vi "EnterDUTInfo.vi"(0 "Enable":bool=TRUE, 5 "error in (no error)":errorcluster, 6 "InputData":string="Enter DUT INFO", 7 "Leidos_sn(t)":bool) -> (10 "DUT INFO":string, 12 "MFR":string, 13 "Desc":string, 14 "SN":string, 15 "LotID":string, 16 "Revision":string, 17 "RaGE PN":string, 18 "OK":bool, 19 "error out":errorcluster)   [LabVIEW 2018]
doc: "Displays a standard dialog box that prompts users to enter information, such as a user name and password.\n--------------------\n\nThis Express VI is configured as follows:\n\nMessage to Display to the User:Enter DUT INFO\nThe inputs are: \nText Entry Box: RaGE PN\nText Entry Box: Revision\nText Entry Box: LotID\nText Entry Box: SN\nText Entry Box: Desc\nText Entry Box: MFR"
panel:
  in  "ESN":string caption="SN"
  out "ESN":string caption="SN"
  in  "MFR":string
  in  "Desc":string
  in  "SN":string
  in  "LotID":string
  in  "Revision":string
  in  "RaGE PN":string
  out "String":string="Enter DUT INFO"
  in  "Cancel":bool
  in  "OK2":bool
  in  "OK1":bool
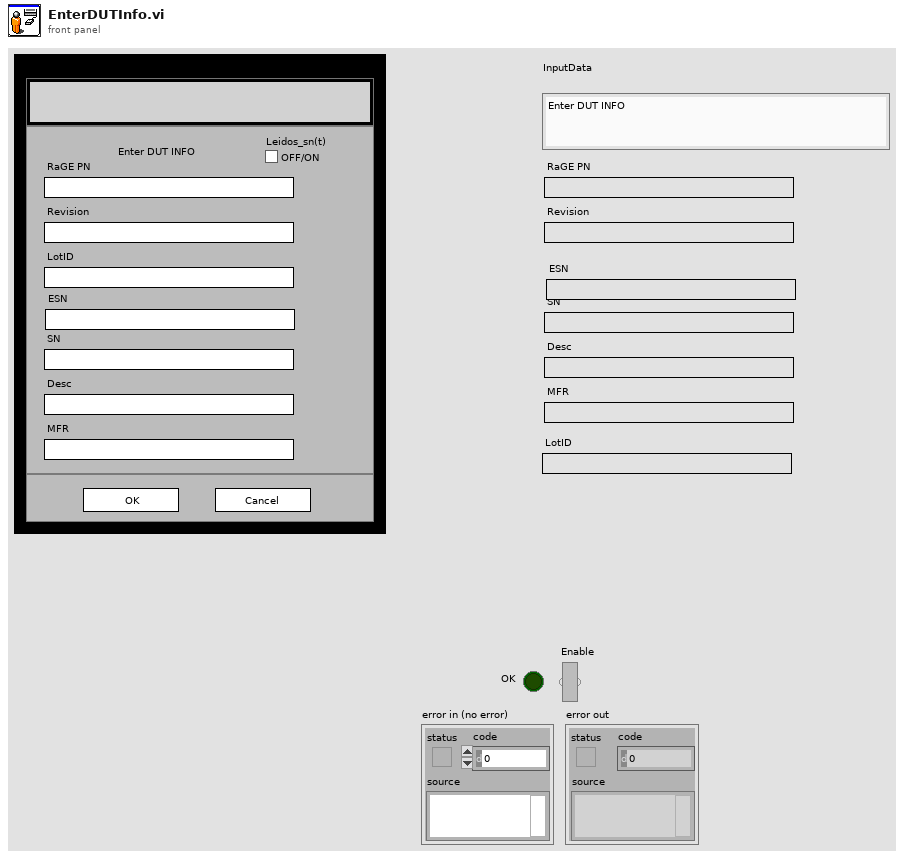
[diagram p1: front panel]
types:
  T1 = enum8{"Enabled", "Disabled", "Disabled and Grayed Out"}
  T2 = cluster{"Input Name":string, "Input Data Type":i32}[]
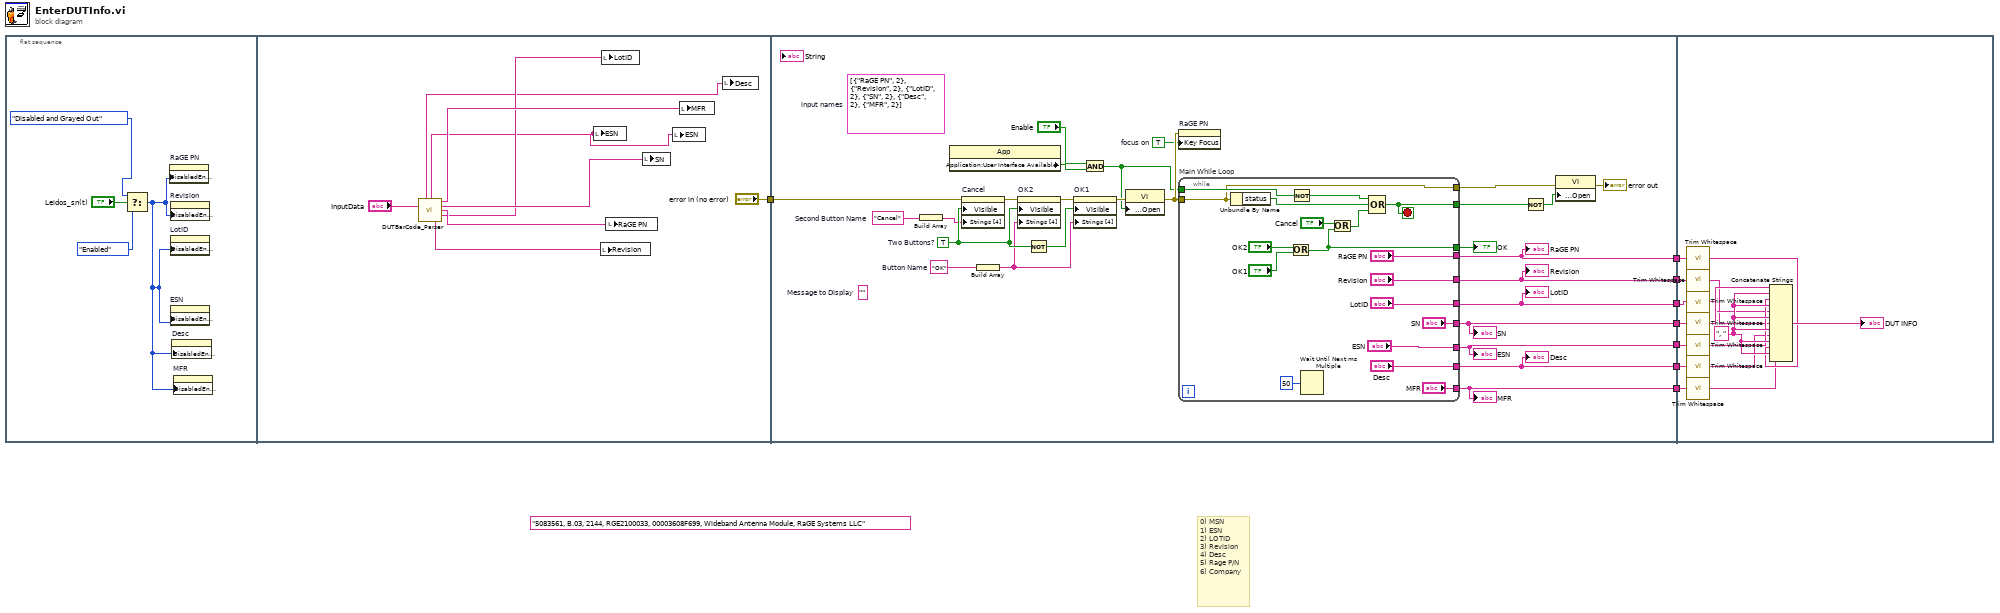
[diagram p0: block diagram]
diagram:
  (unwired) "5083561, B.03, 2144, RGE2100033, 00003608F699, Wideband Antenna Module, RaGE Systems LLC" ("Bar Code")
  # "0) MSN\n1) ESN\n2) LOTID\n3) Revision \n4) Desc\n5) Rage P/N\n6) Company"
  n1 = flat-sequence {
    tunnel: ["error in (no error)"] -> w8
    tunnel: w8 -> [w29]
    tunnel: [w28] -> w7
    tunnel: [w27] -> w6
    tunnel: [w23] -> w5
    tunnel: [w26] -> w4
    tunnel: [w25] -> w3
    tunnel: [w24] -> w2
    tunnel: [w22] -> w1
    tunnel: w7 -> [w82]
    tunnel: w6 -> [w81]
    tunnel: w5 -> [w80]
    tunnel: w4 -> [w79]
    tunnel: w3 -> [w77]
    tunnel: w2 -> [w75]
    tunnel: w1 -> [w74]
    frame #0 {
      n2 = Select(t=T1."Disabled and Grayed Out" ("Disabled"), s="Leidos_sn(t)", f=T1."Enabled" ("Disabled")) -> (s? t:f=w11:T1)
      n3 = property on="RaGE PN" class="Str"("DisabledEnum"=w11) -> ()  [unwired: 2 in, 2 out]
      n4 = property on="Revision" class="Str"("DisabledEnum"=w11) -> ()  [unwired: 2 in, 2 out]
      n5 = property on="LotID" class="Str"("DisabledEnum"=w11) -> ()  [unwired: 2 in, 2 out]
      n6 = property on="ESN" class="Str"("DisabledEnum"=w11) -> ()  [unwired: 2 in, 2 out]
      n7 = property on="Desc" class="Str"("DisabledEnum"=w11) -> ()  [unwired: 2 in, 2 out]
      n8 = property on="MFR" class="Str"("DisabledEnum"=w11) -> ()  [unwired: 2 in, 2 out]
    }
    frame #1 {
      n9 = call "DUTBarCode_Parser.vi"("DUT INFO"="InputData") -> ("Desc"=w14:string, "BC_ESN"=w13:string, "Company"=w19:string, "BC_MSN"=w18:string, "Rage PN"=w17:string, "LotID"=w15:string, "Revision"=w16:string)  [unwired: 5 in, 3 out]
      n10 = local write "ESN"(w13) -> ()
      n11 = local write "Revision"(w16) -> ()
      n12 = local write "LotID"(w15) -> ()
      n13 = local write "RaGE PN"(w17) -> ()
      n14 = local write "SN"(w18) -> ()
      n15 = local write "ESN"(w13) -> ()
      n16 = local write "MFR"(w19) -> ()
      n17 = local write "Desc"(w14) -> ()
    }
    frame #2 {
      w30 = TRUE  # focus on
      (unwired) T2 [{"Input Name"="RaGE PN", "Input Data Type"=2}, {"Input Name"="Revision", "Input Data Type"=2}, {"Input Name"="LotID", "Input Data Type"=2}, {"Input Name"="SN", "Input Data Type"=2}, {"Input Name"="Desc", "Input Data Type"=2}, {"Input Name"="MFR", "Input Data Type"=2}]  # input names
      w40 = "Cancel"  # Second Button Name
      w38 = "OK"  # Button Name
      (unwired) ""  # Message to Display
      w48 = TRUE  # Two Buttons?
      n18 = Build Array(w40) -> (w41:string[])
      n19 = property class="App"() -> ("Application:User Interface Available"=w31:bool)  [unwired: 2 in, 2 out]
      n20 = property on="Cancel" class="Bool"(error in=w29, "Visible"=w48, "Strings [4]"=w41) -> (error out=w45:errorcluster)  [unwired: 1 in, 1 out]
      n21 = Build Array(w38) -> (w39:string[])
      n22 = property on="OK2" class="Bool"(error in=w45, "Visible"=w48, "Strings [4]"=w39) -> (error out=w44:errorcluster)  [unwired: 1 in, 1 out]
      n23 = Not(x=w48) -> (.not. x?=w46:bool)
      n24 = property on="OK1" class="Bool"(error in=w44, "Visible"=w46, "Strings [4]"=w39) -> (error out=w37:errorcluster)  [unwired: 1 in, 1 out]
      n25 = And(x="Enable", y=w31) -> (x .and. y?=w32:bool)
      n26 = property class="VI"(error in=w37, "Front Panel Window:Open"=w32) -> (error out=w36:errorcluster)  [unwired: 1 in, 1 out]
      n27 = property on="RaGE PN" class="Str"(error in=w36, "Key Focus"=w30) -> ()  [unwired: 1 in, 2 out]
      n28 = while "Main While Loop" {
        tunnel: [w63] -> w47
        tunnel: w32 -> [w61]
        tunnel: [w59] -> w42
        tunnel: w36 -> [w58]
        tunnel: [w58] -> w35
        tunnel: ["RaGE PN"] -> w28
        tunnel: ["Revision"] -> w27
        tunnel: ["LotID"] -> w24
        tunnel: ["SN"] -> w22
        tunnel: ["Desc"] -> w26
        tunnel: ["MFR"] -> w25
        tunnel: ["ESN"] -> w23
        stop <- w59 stop-if-true
        n29 = Unbundle By Name(w58) -> ("status"=w56:bool)
        n30 = Or(x="OK2", y="OK1") -> (x .or. y?=w63:bool)
        n31 = Not(x=w61) -> (.not. x?=w60:bool)
        n32 = Wait Until Next ms Multiple(millisecond multiple=u32 50) -> ()  [unwired: 1 out]
        n33 = Or(x="Cancel", y=w63) -> (x .or. y?=w57:bool)
        n34 = Compound Arithmetic op=OR(w60, w56, w57) -> (w59:bool)
      }
      "OK" <- w47
      "RaGE PN" <- w28
      "Revision" <- w27
      "LotID" <- w24
      "SN" <- w22
      "Desc" <- w26
      "MFR" <- w25
      "ESN" <- w23
      n35 = Not(x=w42) -> (.not. x?=w43:bool)
      n36 = property class="VI"(error in=w35, "Front Panel Window:Open"=w43) -> (error out=→"error out":errorcluster)  [unwired: 1 in, 1 out]
    }
    frame #3 {
      w78 = ", " ("string")
      n37 = call <vilib>:"Trim Whitespace.vi"("string"=w82) -> ("trimmed string"=w68:string)  [unwired: 1 in]
      n38 = call <vilib>:"Trim Whitespace.vi"("string"=w81) -> ("trimmed string"=w70:string)  [unwired: 1 in]
      n39 = call <vilib>:"Trim Whitespace.vi"("string"=w75) -> ("trimmed string"=w71:string)  [unwired: 1 in]
      n40 = call <vilib>:"Trim Whitespace.vi"("string"=w74) -> ("trimmed string"=w73:string)  [unwired: 1 in]
      n41 = call <vilib>:"Trim Whitespace.vi"("string"=w80) -> ("trimmed string"=w72:string)  [unwired: 1 in]
      n42 = call <vilib>:"Trim Whitespace.vi"("string"=w79) -> ("trimmed string"=w69:string)  [unwired: 1 in]
      n43 = call <vilib>:"Trim Whitespace.vi"("string"=w77) -> ("trimmed string"=w67:string)  [unwired: 1 in]
      n44 = Concatenate Strings(w73, w78, w72, w78, w71, w78, w70, w78, w69, w78, w68, w78, w67) -> (→"DUT INFO":string)
    }
  }
